vi "Power ON all drivers.vi"(8 "error in (no error)":errorcluster, 11 "Conections in":T1) -> (0 "error out":errorcluster, 3 "Conections out":T1)   [LabVIEW 2017]
uses:
  ctl/connections.ctl
  <vilib>/addons/eal4LabVIEW/eal4LabVIEW.lvlib
  Servo drive module.lvlib
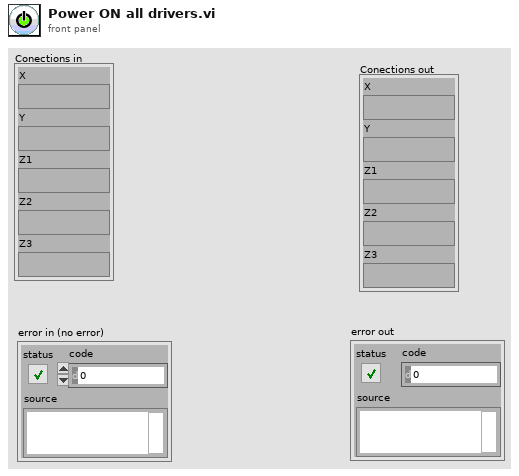
[diagram p1: front panel]
types:
  T1 = typedef "Servo drive module.lvlib/connections.ctl" = cluster{"X":variant, "Y":variant, "Z1":variant, "Z2":variant, "Z3":variant}
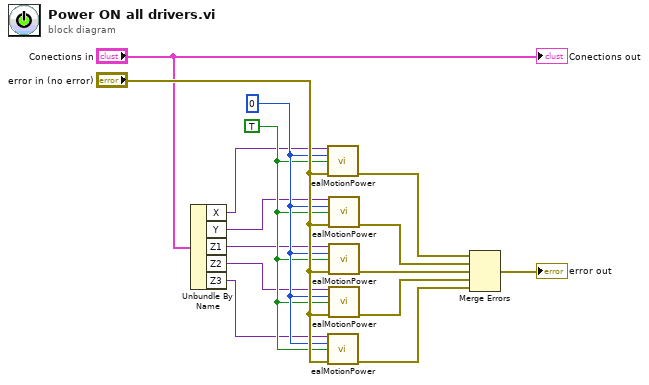
[diagram p0: block diagram]
diagram:
  w9 = 0
  w8 = TRUE ("value")
  n1 = Unbundle By Name("Conections in") -> ("X"=w3:variant, "Y"=w4:variant, "Z1"=w5:variant, "Z2"=w6:variant, "Z3"=w7:variant)
  n2 = call <vilib>:"ealMotionPower.vi"("connection in"=w3, "slave index"=w9, "value"=w8, "error in (no error)"="error in (no error)") -> ("error out"=w11:errorcluster)  [unwired: 10 in, 1 out]
  n3 = call <vilib>:"ealMotionPower.vi"("connection in"=w7, "slave index"=w9, "value"=w8, "error in (no error)"="error in (no error)") -> ("error out"=w15:errorcluster)  [unwired: 10 in, 1 out]
  n4 = call <vilib>:"ealMotionPower.vi"("connection in"=w4, "slave index"=w9, "value"=w8, "error in (no error)"="error in (no error)") -> ("error out"=w12:errorcluster)  [unwired: 10 in, 1 out]
  n5 = call <vilib>:"ealMotionPower.vi"("connection in"=w5, "slave index"=w9, "value"=w8, "error in (no error)"="error in (no error)") -> ("error out"=w13:errorcluster)  [unwired: 10 in, 1 out]
  n6 = call <vilib>:"ealMotionPower.vi"("connection in"=w6, "slave index"=w9, "value"=w8, "error in (no error)"="error in (no error)") -> ("error out"=w14:errorcluster)  [unwired: 10 in, 1 out]
  n7 = Merge Errors(w11, w12, w13, w14, w15) -> (→"error out":errorcluster)
  "Conections out" <- "Conections in"
